vi "test_Add Command_Use SysDef with Command with MetaData Channels.vi"(8 "error in (no error)":errorcluster, 11 "TestCase in":refnum<class "Instrument Addon Scripting API Messages Unit Tests.lvclass">) -> (0 "error out":errorcluster, 3 "TestCase out":refnum<class "Instrument Addon Scripting API Messages Unit Tests.lvclass">)   [LabVIEW 2018, in "Instrument Addon Scripting API Messages Unit Tests.lvclass"]
uses:
  Instrument Addon Scripting API Messages Unit Tests.lvclass
  APIs/Scripting API/TypeDefs/Command Settings.ctl
  <vilib>/NI Veristand/Custom Device API/Custom Device Item Ref.ctl
  APIs/Scripting API/TypeDefs/Padding.ctl
  Addon/Addon Shared/Types/Command Parameters.ctl
  Addon/Addon Shared/Types/Linked Channel Cluster.ctl
  Addon/Addon Shared/Types/FG Control.ctl
  Instrument Addon Scripting API Messages Unit Tests.lvclass/Instrument Addon Scripting API Messages Unit Tests.ctl
  Addon/Addon Shared/SubVIs/Constants.vi
  <vilib>/NI/NI VeriStand Advanced SysDef API/_SubVIs/SysDef.Search.GUID.vi
  <vilib>/NI Veristand/Custom Device API/NI VeriStand - Get Item Property.vi
  <vilib>/NI Veristand/Custom Device API/Get Item Property (String).vi
  <vilib>/NI Veristand/Custom Device API/Get Item Property (String Array).vi
  <vilib>/NI Veristand/Custom Device API/Get Item Property (Boolean).vi
  <vilib>/NI Veristand/Custom Device API/Get Item Property (U32).vi
  <vilib>/NI Veristand/Custom Device API/NI VeriStand - Set Item Property.vi
  <vilib>/NI Veristand/Custom Device API/Set Item Property (String).vi
  <vilib>/NI Veristand/Custom Device API/Set Item Property (String Array).vi
  <vilib>/NI Veristand/Custom Device API/Set Item Property (Boolean).vi
  <vilib>/NI Veristand/Custom Device API/Set Item Property (U32).vi
  <vilib>/addons/_JKI Toolkits/VI Tester/TestCase.llb/TestCase.lvclass
  Instrument Addon Scripting API Test Assets/Instrument Addon Scripting API Test Assets.lvclass
  APIs/Scripting API/Instrument Addon Scripting API.lvlib
  Addon/Addon Shared/Instrument Addon Shared.lvlib
  <vilib>/NI/NI VeriStand Advanced SysDef API/SysDef API/Advanced System Definition.lvlib
  <vilib>/NI Veristand/Custom Device API/Custom Device API.lvlib
  C:/Program Files (x86)/National Instruments/LabVIEW 2018/vi.lib/addons/_JKI Toolkits/VI Tester/TestCase.llb/TestCase.lvclass
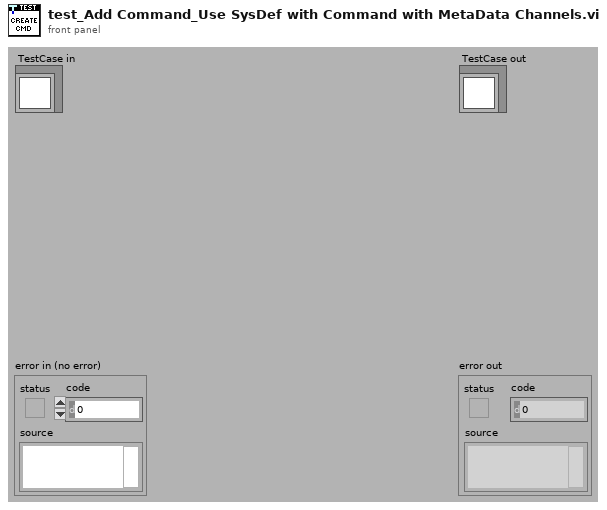
[diagram p1: front panel]
types:
  T1 = typedef "Instrument Addon Shared.lvlib/FG Control.ctl" = enum16{"Get", "Set"}
  T2 = typedef "Custom Device API.lvlib/Custom Device Item Ref.ctl" = u64
  T3 = cluster{"Variable Name":string, "Channel Ref in":T2}[]
  T4 = typedef "Instrument Addon Scripting API.lvlib/Command Settings.ctl" = cluster{"Command Format":string, "Linked Channels":cluster{"Variable Name":string, "Channel Ref in":T2}[], "Use Padding?":bool, "Padding":T5}
  T5 = typedef "Instrument Addon Scripting API.lvlib/Padding.ctl" = cluster{"Pad Value":u8, "Length":u32}
  T6 = typedef "Instrument Addon Shared.lvlib/Command Parameters.ctl" = cluster{"Command":string, "Linked Channels":T7[], "Pad":bool, "Length":u32, "Pad Value":u8}
  T7 = typedef "Instrument Addon Shared.lvlib/Linked Channel Cluster.ctl" = cluster{"Variable Name":string, "GUID":string}
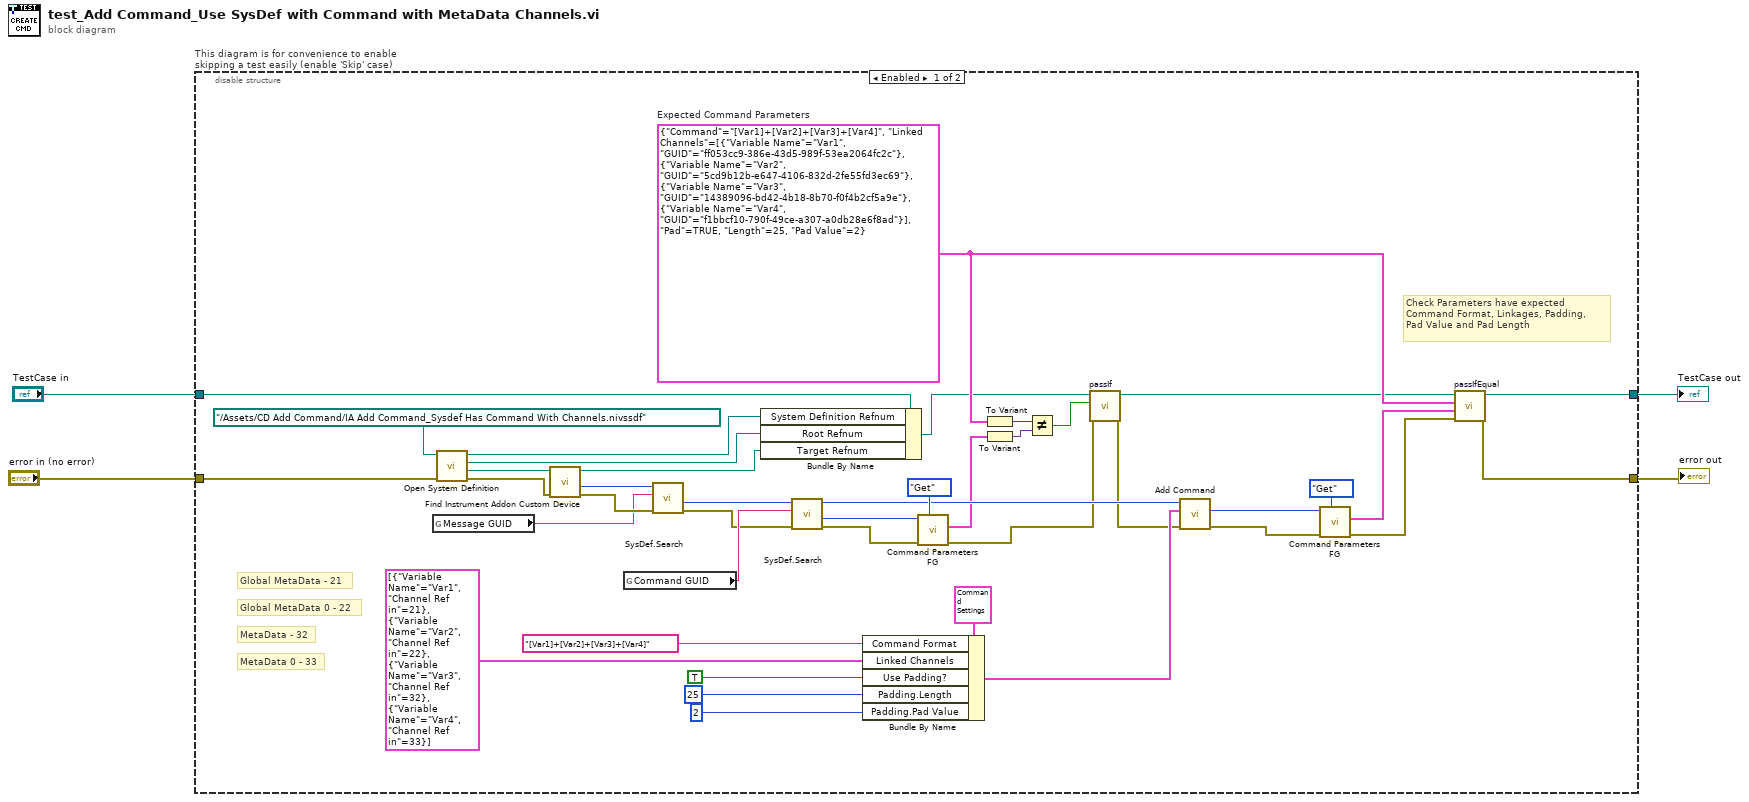
[diagram p0: block diagram]
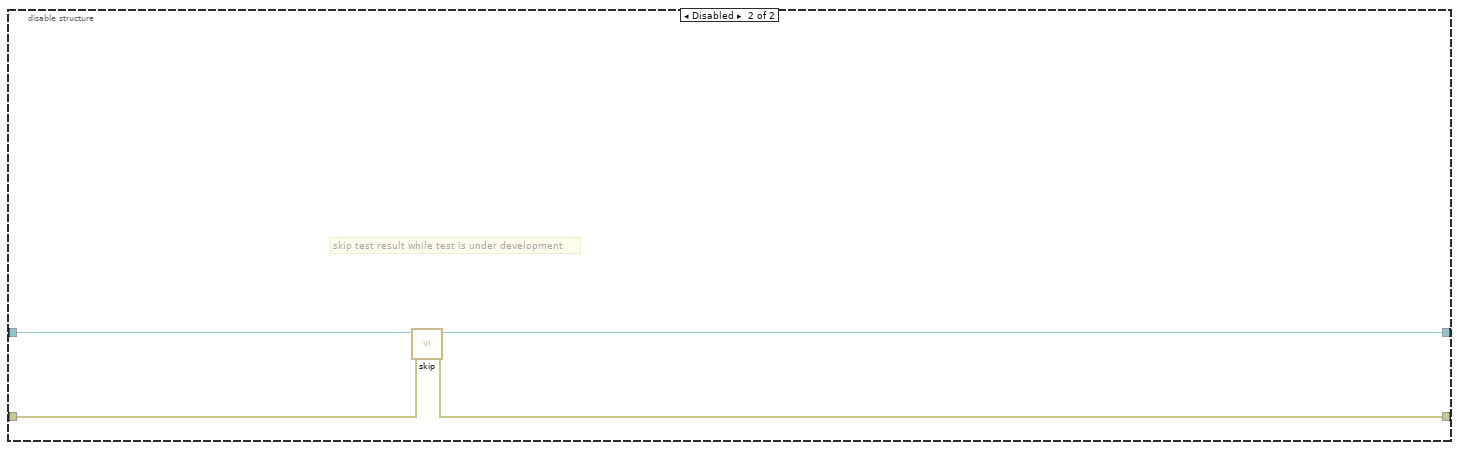
[diagram p2: hidden frame]
diagram:
  n1 = disable-structure "This diagram is for convenience to enable skipping a test easily (enable 'Skip' case)" shown="Enabled" {
    disable-tunnel: "TestCase in" -> [w9 w49]
    disable-tunnel: [w42 w47] -> w1
    disable-tunnel: [w43 w48] -> w3
    disable-tunnel: "error in (no error)" -> [w44 w46]
    frame Enabled {
      w13 = T6 {"Command"="[Var1]+[Var2]+[Var3]+[Var4]", "Linked Channels"=[{"Variable Name"="Var1", "GUID"="ff053cc9-386e-43d5-989f-53ea2064fc2c"}, {"Variable Name"="Var2", "GUID"="5cd9b12b-e647-4106-832d-2fe55fd3ec69"}, {"Variable Name"="Var3", "GUID"="14389096-bd42-4b18-8b70-f0f4b2cf5a9e"}, {"Variable Name"="Var4", "GUID"="f1bbcf10-790f-49ce-a307-a0db28e6f8ad"}], "Pad"=TRUE, "Length"=25, "Pad Value"=2}  # Expected Command Parameters
      # "Check Parameters have expected \nCommand Format, Linkages, Padding,\nPad Value and Pad Length"
      # "MetaData 0 - 33"
      # "MetaData - 32"
      # "Global MetaData 0 - 22"
      # "Global MetaData - 21"
      n2 = global read "Constants.vi" "Message GUID"() -> (w34:string)
      n3 = call "Open System Definition.vi"("error in (no error)"=w44, "System Definition File"=path "../Assets/CD Add Command/IA Add Command_Sysdef Has Command With Channels.nivssdf" ("SDF file")) -> ("error out"=w36:errorcluster, "Target Refnum"=w37:refnum<k24>, "Root Refnum"=w6:refnum<k24>, "System Definition Refnum"=w7:refnum<k24>)  [unwired: 6 in]
      n4 = call "Find Instrument Addon Custom Device.vi"("error in"=w36, "target in"=w37) -> ("error out"=w35:errorcluster, "NodeID"=w29:u64, "target out"=w5:refnum<k24>)  [unwired: 7 in]
      n5 = global read "Constants.vi" "Command GUID"() -> (w24:string)
      n6 = call-poly <vilib>:"SysDef.Search.vi"("error in (no error)"=w35, "GUID"=w34, "nodeID"=w29) -> ("error out"=w18:errorcluster, "Value out"=w20:u64)  [unwired: 5 in, 2 out]
      n7 = Bundle By Name(cluster=w9, "System Definition Refnum"=w7, "Root Refnum"=w6, "Target Refnum"=w5) -> (w8:refnum<class "Instrument Addon Scripting API Messages Unit Tests.lvclass">)
      n8 = call-poly <vilib>:"SysDef.Search.vi"("error in (no error)"=w18, "GUID"=w24, "nodeID"=w20) -> ("error out"=w22:errorcluster, "Value out"=w23:u64, "nodeID out"=w19:u64)  [unwired: 5 in, 1 out]
      n9 = Bundle By Name(cluster=T4 {"Command Format"="[Var1]+[Var2]", "Linked Channels"=[{"Variable Name"="Var1", "Channel Ref in"=32}, {"Variable Name"="Var2", "Channel Ref in"=33}], "Use Padding?"=FALSE, "Padding"={"Pad Value"=0, "Length"=0}} ("Settings"), "Command Format"="[Var1]+[Var2]+[Var3]+[Var4]", "Linked Channels"=T3 [{"Variable Name"="Var1", "Channel Ref in"=21}, {"Variable Name"="Var2", "Channel Ref in"=22}, {"Variable Name"="Var3", "Channel Ref in"=32}, {"Variable Name"="Var4", "Channel Ref in"=33}], "Use Padding?"=TRUE ("Pad"), "Padding.Length"=u32 25, "Padding.Pad Value"=u8 2) -> (w32:T4)
      n10 = call "Command Parameters FG.vi"("Action"=FG_Control."Get", "error in (no error)"=w22, "Item Ref in"=w23) -> ("error out"=w12:errorcluster, "Command Parameters"=w14:T6)  [unwired: 6 in, 1 out]
      n11 = To Variant(anything=w13) -> (Variant=w17:variant)
      n12 = To Variant(anything=w14) -> (Variant=w16:variant)
      n13 = Not Equal?(x=w17, y=w16) -> (x != y?=w15:bool)
      n14 = call-dynamic "passIf.vi"("error in (no error)"=w12, "pass"=w15, "TestCase in"=w8) -> ("error out"=w11:errorcluster, "TestCase out"=w10:refnum<class "Instrument Addon Scripting API Messages Unit Tests.lvclass">)  [unwired: 7 in]
      n15 = call "Add Command.vi"("Error In"=w11, "Settings"=w32, "Message Refnum In"=w19) -> ("Error Out"=w25:errorcluster, "Command Refnum"=w40:T2)  [unwired: 6 in, 1 out]
      n16 = call "Command Parameters FG.vi"("Action"=FG_Control."Get", "error in (no error)"=w25, "Item Ref in"=w40) -> ("error out"=w39:errorcluster, "Command Parameters"=w38:T6)  [unwired: 6 in, 1 out]
      n17 = call-dynamic "passIfEqual.vi"("error in (no error)"=w39, "y"=w38, "x"=w13, "TestCase in"=w10) -> ("error out"=w43:errorcluster, "TestCase out"=w42:refnum<class "Instrument Addon Scripting API Messages Unit Tests.lvclass">)  [unwired: 6 in]
    }
    frame Disabled {
      # "skip test result while test is under development"
      n18 = call <vilib>:"skip.vi"("error in (no error)"=w46, "TestCase in"=w49) -> ("error out"=w48:errorcluster, "TestCase out"=w47:refnum<class "Instrument Addon Scripting API Messages Unit Tests.lvclass">)  [unwired: 8 in]
    }
  }
  "error out" <- w3
  "TestCase out" <- w1
